vi "Header Footer Add Cell.vi"(0 "PdfP Table":refnum<k24>, 1 "Header or Footer":T1, 5 "Page #":i32, 7 "Total page #":i32, 9 "Header Footer Cluster with references":T2={"Start page"=1, "Type"=enum."Select", "Start with #"=1, "Alignment"=enum."Center", "Vertical Alignement"=enum."MIDDLE", "Page #"={"Text 1"="", "Text 2"="", "Text 3"=""}, "Text"=refnum, "Scaled Img"=refnum, "PdfPCell"=refnum, "PdfPTable"=refnum, "Font Cluster"={"Name"="", "Size"=-1.0, "Color"=0, "Style"={"Bold"=FALSE, "Italic"=FALSE, "Underline"=FALSE, "Strikeout"=FALSE}, "Type"={"Type&direction"=enum."Select", "Embedded"=FALSE, "Encoding"=""}}, "Font "=refnum, "Img (%)"=100.0, "Line"={"Line"=enum."Horizontal line", "Thickness (points)"=0.75, "Colour"=7171459}, "Line spacing"=enum."Select"}, 11 "error in (no error)":errorcluster) -> (4 "PdfP Table duplicate":refnum<k24>, 15 "error out":errorcluster)   [LabVIEW 2020, in "Exaprom PDF.lvlib"]
doc: "Version 1.0\nDeveloped by Jean-Marc Simard\nCopyright © 2010, Exaprom Inc.\nAll rights reserved.\nLicense: BSD\n\nWith iTextSharp 4.1.6 (http://itextsharp.sourceforge.net)\nunder Mozilla Public License Version 1.1\n(http://www.mozilla.org/MPL/MPL-1.1.html)"
uses:
  <userlib>/labview-PDF-writer-master/Exaprom PDF.lvlib
  C:/Program Files (x86)/National Instruments/LabVIEW 2020/user.lib/labview-PDF-writer-master/DLL/itextsharp.dll
  DLL/itextsharp.dll
  <userlib>/labview-PDF-writer-master/Controls/Header, Footer and Watermark Controls/Header Footer Cluster with references.ctl
  <userlib>/labview-PDF-writer-master/Controls/Header, Footer and Watermark Controls/Header Footer Type.ctl
  <userlib>/labview-PDF-writer-master/Controls/Header, Footer and Watermark Controls/Header footer horiz alignment.ctl
  <userlib>/labview-PDF-writer-master/Controls/Table Controls/Cell Vertical alignment.ctl
  <userlib>/labview-PDF-writer-master/Controls/Header, Footer and Watermark Controls/Page number.ctl
  <userlib>/labview-PDF-writer-master/Controls/Font Controls/Font complete cluster horizontal.ctl
  <userlib>/labview-PDF-writer-master/Controls/Font Controls/Font size.ctl
  <userlib>/labview-PDF-writer-master/Controls/Font Controls/Font color.ctl
  <userlib>/labview-PDF-writer-master/Controls/Font Controls/Type and encoding.ctl
  <userlib>/labview-PDF-writer-master/Controls/Text Controls/Unicode/Type and run direction.ctl
  <userlib>/labview-PDF-writer-master/Controls/Header, Footer and Watermark Controls/Header Footer Line.ctl
  <userlib>/labview-PDF-writer-master/Controls/Text Controls/Line spacing.ctl
  <userlib>/labview-PDF-writer-master/Controls/Header, Footer and Watermark Controls/Header or Footer.ctl
  <userlib>/labview-PDF-writer-master/Controls/Font Controls/Font complete cluster.ctl
  <userlib>/labview-PDF-writer-master/LV Class/Fonts Class/Font Class.lvclass
panel:
  # "X"
  # "Y"
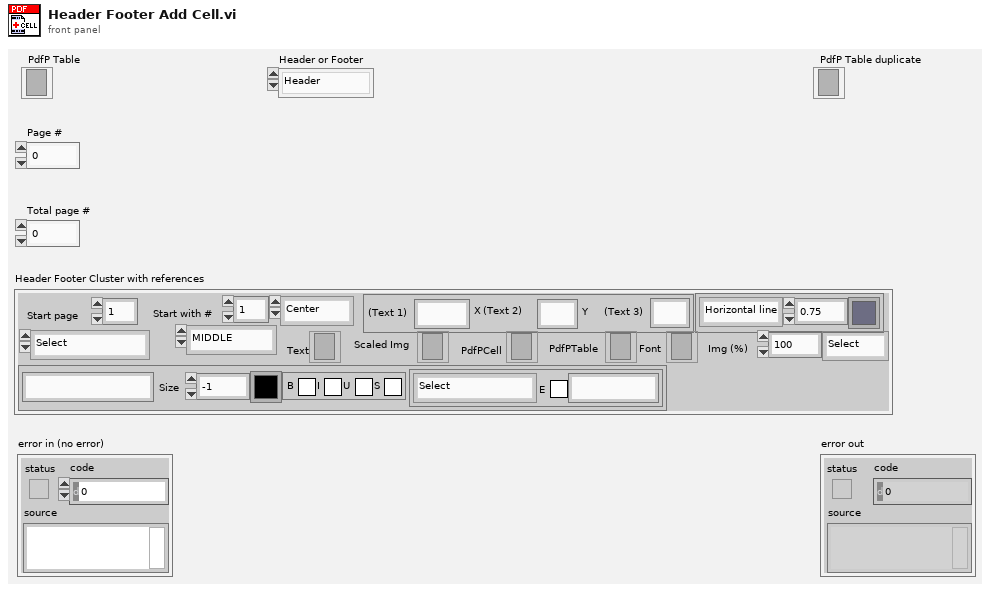
[diagram p1: front panel]
types:
  T1 = typedef "Exaprom PDF.lvlib/Header or Footer.ctl" = enum16{"Header", "Footer"}
  T2 = typedef "Exaprom PDF.lvlib/Header Footer Cluster with references.ctl" = cluster{"Start page":i32, "Type":T3, "Start with #":i32, "Alignment":T4, "Vertical Alignement":T5, "Page #":T6, "Text":refnum<k24>, "Scaled Img":refnum<k24>, "PdfPCell":refnum<k24>, "PdfPTable":refnum<k24>, "Font Cluster":T7, "Font ":refnum<k24>, "Img (%)":sgl, "Line":cluster{"Line":T12, "Thickness (points)":sgl, "Colour":T9}, "Line spacing":T13}
  T3 = typedef "Exaprom PDF.lvlib/Header Footer Type.ctl" = enum16{"Select", "Text", "Text + hyperlink", "Page number", "Image", "Image + hyperlink"}
  T4 = typedef "Exaprom PDF.lvlib/Header footer horiz alignment.ctl" = enum16{"Left", "Center", "Right"}
  T5 = typedef "Exaprom PDF.lvlib/Cell Vertical alignment.ctl" = enum16{"TOP", "MIDDLE", "BOTTOM"}
  T6 = typedef "Exaprom PDF.lvlib/Page number.ctl" = cluster{"Text 1":string, "Text 2":string, "Text 3":string}
  T7 = typedef "Exaprom PDF.lvlib/Font complete cluster horizontal.ctl" = cluster{"Name":string, "Size":T8, "Color":T9, "Style":cluster{"Bold":bool, "Italic":bool, "Underline":bool, "Strikeout":bool}, "Type":T10}
  T8 = typedef "Exaprom PDF.lvlib/Font size.ctl" = sgl
  T9 = typedef "Exaprom PDF.lvlib/Font color.ctl" = u32
  T10 = typedef "Exaprom PDF.lvlib/Type and encoding.ctl" = cluster{"Type&direction":T11, "Embedded":bool, "Encoding":string}
  T11 = typedef "Exaprom PDF.lvlib/Type and run direction.ctl" = enum16{"Select", "ASCII", "UTF-16", "UTF-16 (default)", "UTF-16 (LTR)", "UTF-16 (RTL)"}
  T12 = typedef "Exaprom PDF.lvlib/Header Footer Line.ctl" = enum16{"No line", "Horizontal line"}
  T13 = typedef "Exaprom PDF.lvlib/Line spacing.ctl" = enum16{"Select", "1.0", "1.5", "2.0"}
  T14 = typedef "Exaprom PDF.lvlib/Font complete cluster.ctl" = cluster{"Name":string, "Size":T8, "Color":T9, "Style":cluster{"Bold":bool, "Italic":bool, "Underline":bool, "Strikeout":bool}, "Type":T10}
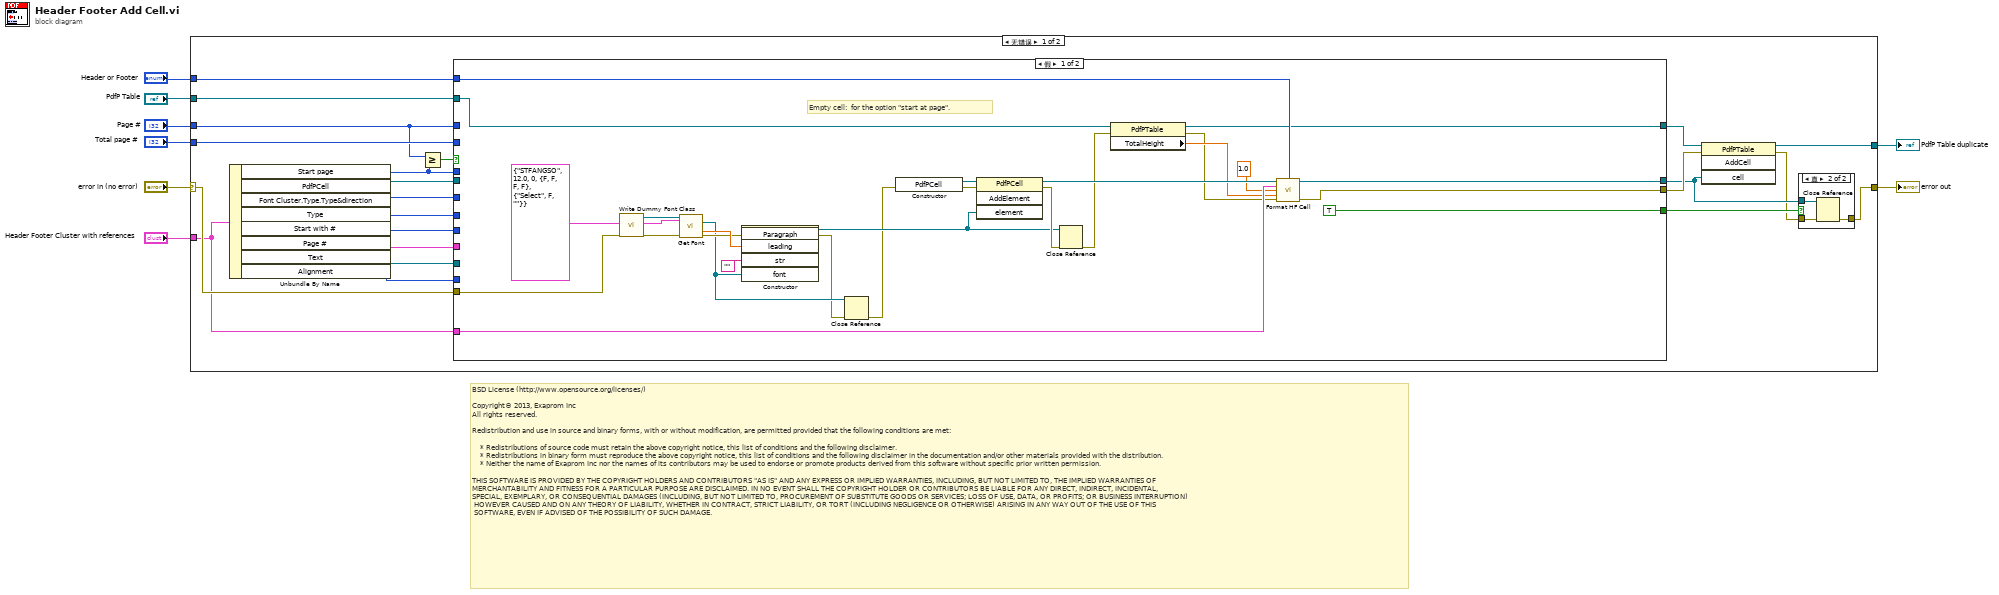
[diagram p0: block diagram]
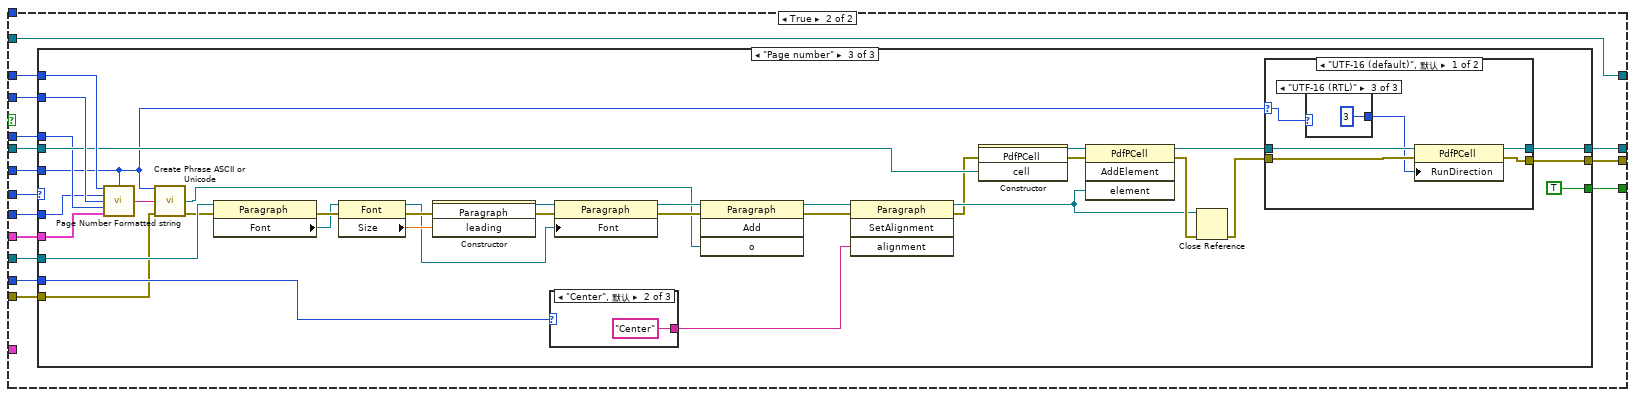
[diagram p2: hidden frame]
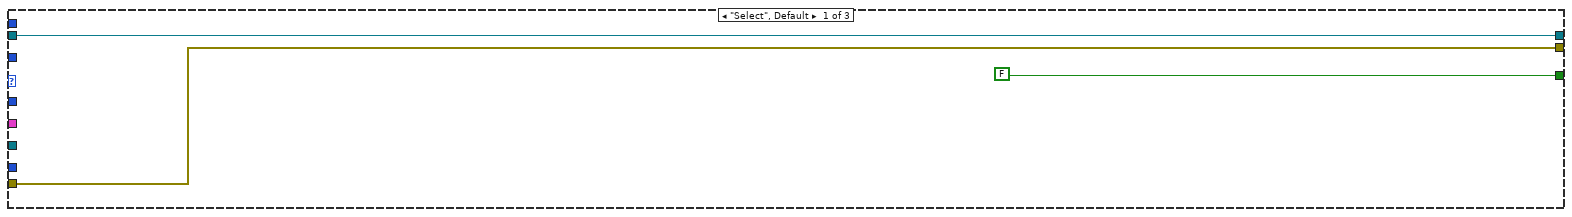
[diagram p3: hidden frame]
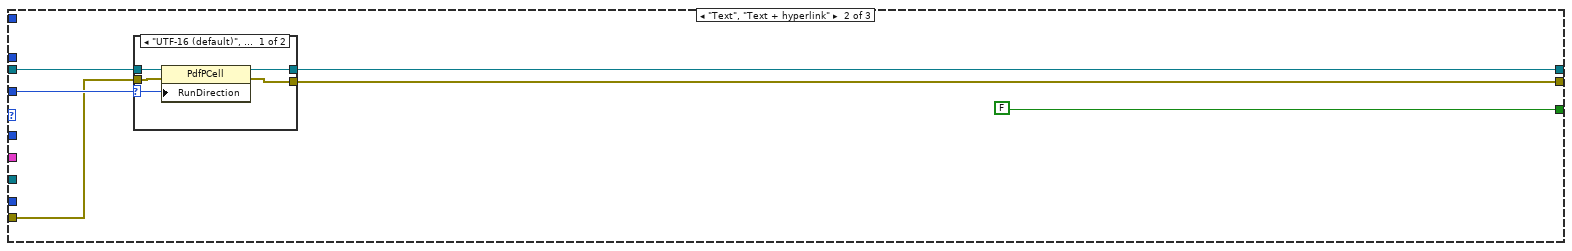
[diagram p4: hidden frame]
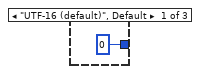
[diagram p6: hidden frame]
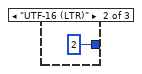
[diagram p7: hidden frame]
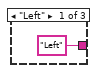
[diagram p9: hidden frame]
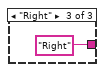
[diagram p10: hidden frame]
diagram:
  # "BSD License (http://www.opensource.org/licenses/)\n\nCopyright© 2013, Exaprom Inc\nAll rights reserved.\n\nRedistribution and use in source and binary forms, with or without modification, are permitted provided that the following conditions are met:\n\n    * Redistributions of source code must retain the above copyright notice, this list of conditions and the following disclaimer.\n    * Redistributions in binary form must reproduce the above copyright notice, this list of conditions and the following disclaimer in the documentation and/or other materials provided with the distribution.\n    * Neither the name of Exaprom Inc nor the names of its contributors may be used to endorse or promote products derived from this software without specific prior written permission.\n\nTHIS SOFTWARE IS PROVIDED BY THE COPYRIGHT HOLDERS AND CONTRIBUTORS \"AS IS\" AND ANY EXPRESS OR IMPLIED WARRANTIES, INCLUDING, BUT NOT LIMITED TO, THE IMPLIED WARRANTIES OF \nMERCHANTABILITY AND FITNESS FOR A PARTICULAR PURPOSE ARE DISCLAIMED. IN NO EVENT SHALL THE COPYRIGHT HOLDER OR CONTRIBUTORS BE LIABLE FOR ANY DIRECT, INDIRECT, INCIDENTAL,\nSPECIAL, EXEMPLARY, OR CONSEQUENTIAL DAMAGES (INCLUDING, BUT NOT LIMITED TO, PROCUREMENT OF SUBSTITUTE GOODS OR SERVICES; LOSS OF USE, DATA, OR PROFITS; OR BUSINESS INTERRUPTION)\n HOWEVER CAUSED AND ON ANY THEORY OF LIABILITY, WHETHER IN CONTRACT, STRICT LIABILITY, OR TORT (INCLUDING NEGLIGENCE OR OTHERWISE) ARISING IN ANY WAY OUT OF THE USE OF THIS\n SOFTWARE, EVEN IF ADVISED OF THE POSSIBILITY OF SUCH DAMAGE."
  n1 = case shown="无错误" "error in (no error)" {
    selector: "error in (no error)" -> [w26 w142]
    tunnel: "Header Footer Cluster with references" -> [w25 _]
    tunnel: "Page #" -> [w22 _]
    tunnel: "Total page #" -> [w27 _]
    tunnel: [w16 w142] -> w5
    tunnel: [w29 w141] -> w2
    tunnel: "PdfP Table" -> [w19 w141]
    tunnel: "Header or Footer" -> [w20 _]
    frame No Error {
      n2 = Unbundle By Name(w25) -> ("Start page"=w15:i32, "PdfPCell"=w23:refnum<k24>, "Font Cluster.Type.Type&direction"=w13:T11, "Type"=w14:T3, "Start with #"=w10:i32, "Page #"=w9:T6, "Text"=w11:refnum<k24>, "Alignment"=w12:T4)
      n3 = Greater Or Equal?(x=w22, y=w15) -> (x >= y?=w21:bool)
      n4 = case shown="假" w21 {
        tunnel: [w42 w71] -> w30
        tunnel: [w43 w70] -> w28
        tunnel: w27 -> [_ w69]
        tunnel: w26 -> [w31 w68]
        tunnel: w25 -> [w40 _]
        tunnel: [TRUE w67] -> w24
        tunnel: w14 -> [_ w63]
        tunnel: w23 -> [_ w66]
        tunnel: w22 -> [_ w65]
        tunnel: w20 -> [w41 _]
        tunnel: w19 -> [w38 w64]
        tunnel: [w36 w64] -> w18
        tunnel: w15 -> [_ w62]
        tunnel: w13 -> [_ w61]
        tunnel: w12 -> [_ w60]
        tunnel: w11 -> [_ w59]
        tunnel: w10 -> [_ w58]
        tunnel: w9 -> [_ w57]
        frame False {
          # "Empty cell:  for the option \"start at page\"."
          n5 = call <userlib>:"Write Dummy Font Class.vi"("error in (no error)"=w31) -> ("Font OUT"=w32:refnum<class "Font Class.lvclass">, "error out"=w33:errorcluster)  [unwired: 13 in]
          n6 = call <userlib>:"Get Font.vi"("Font"=w32, "Font IN"=T14 {"Name"="STFANGSO", "Size"=12.0, "Color"=0, "Style"={"Bold"=FALSE, "Italic"=FALSE, "Underline"=FALSE, "Strikeout"=FALSE}, "Type"={"Type&direction"=enum."Select", "Embedded"=FALSE, "Encoding"=""}}, "error in (no error)"=w33) -> ("Font"=w47:refnum<k24>, "Font Size"=w51:T8, "error out"=w48:errorcluster)  [unwired: 8 in, 2 out]
          n7 = constructor class="Paragraph"(error in=w48, "leading"=w51, "str"="", "font"=w47) -> (reference out=w52:refnum<k24>, error out=w46:errorcluster)  [unwired: 2 in, 4 out]
          n8 = Close Reference(reference=w47, error in (no error)=w46) -> (error out=w45:errorcluster)
          n9 = constructor class="PdfPCell"(error in=w45) -> (reference out=w54:refnum<k24>, error out=w53:errorcluster)  [unwired: 2 in, 1 out]
          n10 = invoke class="PdfPCell" method="AddElement"(reference=w54, error in=w53, "element"=w52) -> (reference out=w44:refnum<k24>, error out=w55:errorcluster)  [unwired: 1 in, 2 out]
          n11 = Close Reference(reference=w52, error in (no error)=w55) -> (error out=w35:errorcluster)
          n12 = property class="PdfPTable"(reference=w38, error in=w35) -> (reference out=w36:refnum<k24>, error out=w34:errorcluster, "TotalHeight"=w37:sgl)
          n13 = call <userlib>:"Format HF Cell.vi"("PdfP Cell"=w44, "Header or Footer"=w41, "Header Footer Cluster with references"=w40, "Padding (points)"=sgl 1.0 ("FixedHeight (points)"), "FixedHeight (points)"=w37, "error in (no error)"=w34) -> ("PdfP Cell duplicate"=w43:refnum<k24>, "error out"=w42:errorcluster)  [unwired: 8 out]
        }
        frame True {
          n14 = case shown="\"Page number\"" w63 {
            tunnel: w66 -> [w74 w78 w114]
            tunnel: [w74 w77 w92] -> w70
            tunnel: w69 -> [_ _ w122]
            tunnel: w65 -> [_ _ w121]
            tunnel: w68 -> [w73 w75 w103]
            tunnel: [w73 w76 w91] -> w71
            tunnel: [FALSE FALSE TRUE] -> w67
            tunnel: w62 -> [_ _ w109]
            tunnel: w61 -> [_ w79 w88]
            tunnel: w60 -> [_ _ w107]
            tunnel: w59 -> [_ _ w106]
            tunnel: w58 -> [_ _ w105]
            tunnel: w57 -> [_ _ w104]
            frame "Select", Default {
            }
            frame "Text", "Text + hyperlink" {
              n15 = case shown="\"UTF-16 (default)\", 默认" w79 {
                selector: w79 -> [w83 _]
                tunnel: w78 -> [w85 w87]
                tunnel: [w84 w87] -> w77
                tunnel: [w82 w86] -> w76
                tunnel: w75 -> [w81 w86]
                frame "UTF-16 (default)", Default {
                  n16 = property class="PdfPCell"(reference=w85, error in=w81, "RunDirection"=w83) -> (reference out=w84:refnum<k24>, error out=w82:errorcluster)
                }
                frame "ASCII" {
                }
              }
            }
            frame "Page number" {
              n17 = call <userlib>:"Page Number Formatted string.vi"("Page #"=w121, "Character type"=w88, "Start with #"=w105, "Total page #"=w122, "Start at page"=w109, "Page # cluster"=w104) -> ("Page string"=w108:string)  [unwired: 9 out]
              n18 = call <userlib>:"Create Phrase ASCII or Unicode.vi"("Character type"=w88, "Text"=w108, "error in (no error)"=w103) -> ("Phrase refnum"=w93:refnum<k24>, "error out"=w102:errorcluster)  [unwired: 10 in, 1 out]
              n19 = property class="Paragraph"(reference=w106, error in=w102) -> (error out=w119:errorcluster, "Font"=w117:refnum<k24>)  [unwired: 1 out]
              n20 = property class="Font"(reference=w117, error in=w119) -> (reference out=w98:refnum<k24>, error out=w99:errorcluster, "Size"=w118:sgl)
              n21 = constructor class="Paragraph"(error in=w99, "leading"=w118) -> (reference out=w101:refnum<k24>, error out=w100:errorcluster)  [unwired: 2 in, 2 out]
              n22 = case shown="\"Center\", 默认" w107 {
                tunnel: ["Left" "Center" "Right"] -> w116
                frame "Left" {
                }
                frame "Center", Default {
                }
                frame "Right" {
                }
              }
              n23 = property class="Paragraph"(reference=w101, error in=w100, "Font"=w98) -> (reference out=w97:refnum<k24>, error out=w96:errorcluster)
              n24 = invoke class="Paragraph" method="Add"(reference=w97, error in=w96, "o"=w93) -> (reference out=w94:refnum<k24>, error out=w95:errorcluster)  [unwired: 1 in, 2 out]
              n25 = invoke class="Paragraph" method="SetAlignment"(reference=w94, error in=w95, "alignment"=w116) -> (reference out=w115:refnum<k24>, error out=w110:errorcluster)  [unwired: 1 in, 2 out]
              n26 = constructor class="PdfPCell"(error in=w110, "cell"=w114) -> (reference out=w113:refnum<k24>, error out=w111:errorcluster)  [unwired: 2 in, 2 out]
              n27 = invoke class="PdfPCell" method="AddElement"(reference=w113, error in=w111, "element"=w115) -> (reference out=w89:refnum<k24>, error out=w120:errorcluster)  [unwired: 1 in, 2 out]
              n28 = Close Reference(reference=w115, error in (no error)=w120) -> (error out=w90:errorcluster)
              n29 = case shown="\"UTF-16 (default)\", 默认" w88 {
                selector: w88 -> [w124 _]
                tunnel: w89 -> [w128 w133]
                tunnel: [w127 w133] -> w92
                tunnel: [w126 w132] -> w91
                tunnel: w90 -> [w125 w132]
                frame "UTF-16 (default)", Default {
                  n30 = case shown="\"UTF-16 (RTL)\"" w124 {
                    tunnel: [0 ("RunDirection") 2 ("RunDirection") 3 ("RunDirection")] -> w123
                    frame "UTF-16 (default)", Default {
                    }
                    frame "UTF-16 (LTR)" {
                    }
                    frame "UTF-16 (RTL)" {
                    }
                  }
                  n31 = property class="PdfPCell"(reference=w128, error in=w125, "RunDirection"=w123) -> (reference out=w127:refnum<k24>, error out=w126:errorcluster)
                }
                frame "ASCII", "UTF-16" {
                }
              }
            }
          }
        }
      }
      n32 = invoke class="PdfPTable" method="AddCell"(reference=w18, error in=w30, "cell"=w28) -> (reference out=w29:refnum<k24>, error out=w17:errorcluster)  [unwired: 1 in, 2 out]
      n33 = case shown="真" w24 {
        tunnel: w28 -> [_ w140]
        tunnel: w17 -> [w137 w139]
        tunnel: [w137 w138] -> w16
        frame False {
        }
        frame True {
          n34 = Close Reference(reference=w140, error in (no error)=w139) -> (error out=w138:errorcluster)
        }
      }
    }
    frame Error {
    }
  }
  "error out" <- w5
  "PdfP Table duplicate" <- w2
